vi "frw_get_extra_param.vi"(11 "Path":path) -> (2 "extra_string":string, 3 "channels_str":string)   [LabVIEW 2013]
doc: "Reads parameters form EEG file, CSV or EDF"
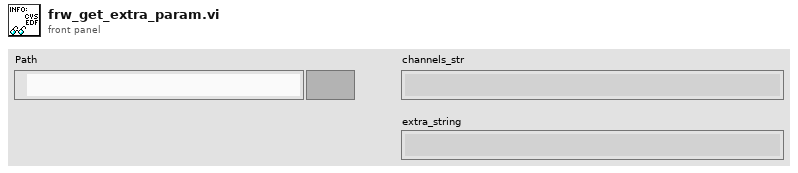
[diagram p1: front panel]
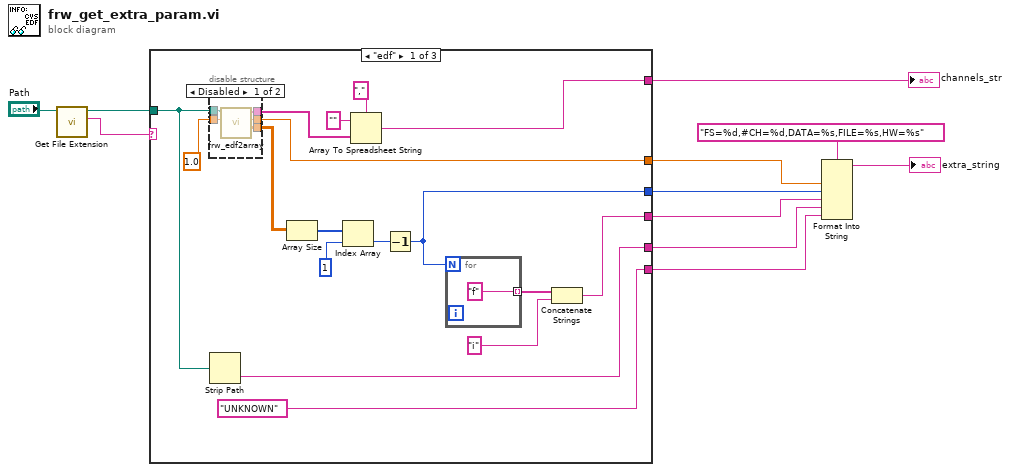
[diagram p0: block diagram]
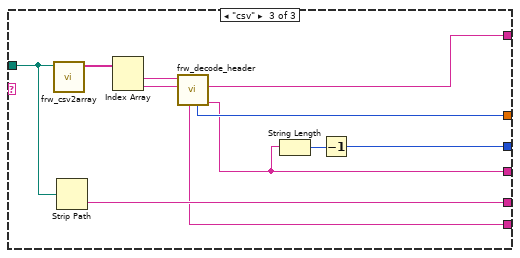
[diagram p4: hidden frame]
diagram:
  n1 = call <vilib>:"Get File Extension.vi"("file"="Path") -> ("lowercase file extension"=w10:string, "dup file"=w9:path)  [unwired: 7 in, 2 out]
  n2 = case shown="\"edf\"" w10 {
    tunnel: w9 -> [w14 _ w37]
    tunnel: [w26 _ w42] -> w8
    tunnel: [w23 _ w41] -> w6
    tunnel: [w15 _ w40] -> w5
    tunnel: [w18 _ w38] -> w4
    tunnel: [w13 _ w36] -> w2
    tunnel: ["UNKNOWN" _ w35] -> w1
    frame "edf" {
      n3 = disable-structure shown="Disabled" {
        disable-tunnel: 1.0 ("block size") -> [w33 _]
        disable-tunnel: [w32 _] -> w24
        disable-tunnel: [w31 _] -> w23
        disable-tunnel: [w30 _] -> w22
        disable-tunnel: w14 -> [w29 _]
        frame Disabled {
          n4 = call "frw_edf2array.vi"("block size (3600s)"=w33, "file path"=w29) -> ("2D array"=w30:dbl[][], "fs"=w31:dbl, "channel names out"=w32:string[])  [unwired: 7 in]
        }
        frame Enabled {
        }
      }
      n5 = Strip Path(path=w14) -> (name=w13:string)  [unwired: 1 out]
      n6 = Array Size(array=w22) -> (size(s)=w21:i32[])
      n7 = Index Array(array=w21, index=1) -> (element=w19:i32)
      n8 = Array To Spreadsheet String(delimiter (Tab)=",", array=w24, 3:"" ("format string")) -> (spreadsheet string=w26:string)
      n9 = Decrement(x=w19) -> (x-1=w18:i32)
      n10 = for {
        N: w18 -> [_]
        tunnel: ["f"] -> w17 mode=indexing
      }
      n11 = Concatenate Strings(w17, "i") -> (w15:string)
    }
    frame Default {
    }
    frame "csv" {
      n12 = call "frw_csv2array.vi"("file path"=w37) -> ("headerarray"=w45:string[])  [unwired: 7 in, 3 out]
      n13 = Strip Path(path=w37) -> (name=w36:string)  [unwired: 1 out]
      n14 = Index Array(array=w45) -> (element #1=w44:string, element #2=w43:string)  [unwired: 2 in]
      n15 = call "frw_decode_header.vi"("header2"=w43, "header1"=w44) -> ("tags"=w40:string, "chLabels"=w42:string, "fs"=w41:i32, "hardware"=w35:string)  [unwired: 4 in, 2 out]
      n16 = String Length(string=w40) -> (length=w39:i32)
      n17 = Decrement(x=w39) -> (x-1=w38:i32)
    }
  }
  "channels_str" <- w8
  n18 = Format Into String(format string="FS=%d,#CH=%d,DATA=%s,FILE=%s,HW=%s", w6, w4, w5, w2, w1) -> (resulting string=→"extra_string":string)  [unwired: 2 in, 1 out]
